vi "GetDVR.vi"(8 "error in":errorcluster, 11 "WindowFrame in":refnum<class "WindowFrame.lvclass">) -> (0 "error out":errorcluster, 2 "dvr":refnum<data-value>, 3 "WindowFrame out":refnum<class "WindowFrame.lvclass">)   [LabVIEW 2021]
uses:
  WindowFrame.lvclass/WindowFrame.ctl
  Data.ctl
  WindowFrame.lvclass
  Action.ctl
  ActionData.ctl
  <vilib>/Utility/miscctls.llb/LVRectTypeDef.ctl
  <vilib>/Utility/miscctls.llb/LVPointTypeDef.ctl
  C:/Users/Dany/OneDrive/LabVIEW/Class/ClassUtilities/ClassByRef/ClassByRef.lvclass
  C:/Users/Dany/OneDrive/LabVIEW/Class/WindowFrame/WindowFrame.lvclass
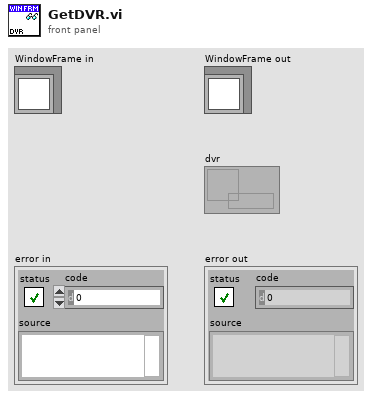
[diagram p1: front panel]
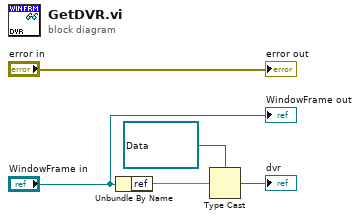
[diagram p0: block diagram]
diagram:
  n1 = Unbundle By Name("WindowFrame in") -> ("ref"=w2)
  n2 = Type Cast(type=refnum<data-value> refnum ("data value reference"), x=w2) -> (*(type *) &x=→"dvr":refnum<data-value>)
  "error out" <- "error in"
  "WindowFrame out" <- "WindowFrame in"
